vi "LeddarRead.vi"(9 "Frame Index":u32, 10 "Connection Mode":enum32{"INIT_FILE", "INIT_LIVE"}(radio), 11 "DeviceControl":refnum<k24>) -> (1 "New Status":bool, 2 "Detections Array":refnum<k24>[](array[refnum]), 3 "DeviceControl Out":refnum<k24>)   [LabVIEW 2012]
uses:
  C:/Program Files/LeddarTech/xtec/LeddarNET2.dll
  Globals.vi
panel:
  out "Timer value":dbl
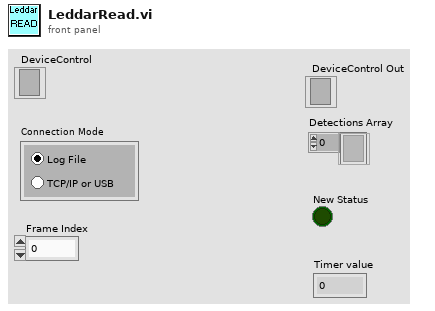
[diagram p1: front panel]
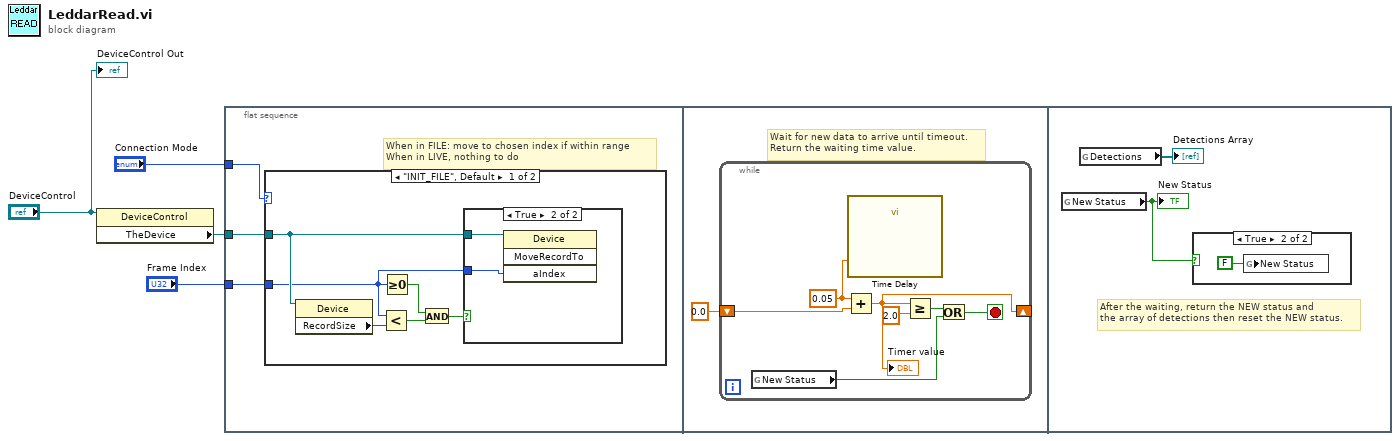
[diagram p0: block diagram]
diagram:
  n1 = property class="DeviceControl"(reference="DeviceControl") -> ("TheDevice"=w2:refnum<k24>)  [unwired: 1 in, 2 out]
  n2 = flat-sequence {
    tunnel: "Connection Mode" -> [w7]
    tunnel: w2 -> [w6]
    tunnel: "Frame Index" -> [w5]
    frame #0 {
      # "When in FILE: move to chosen index if within range\nWhen in LIVE, nothing to do"
      n3 = case shown="\"INIT_FILE\", Default" w7 {
        tunnel: w6 -> [w10 _]
        tunnel: w5 -> [w9 _]
        frame "INIT_FILE", Default {
          n4 = property class="Device"(reference=w10) -> ("RecordSize"=w8:u32)  [unwired: 1 in, 2 out]
          n5 = Less?(x=w9, y=w8) -> (x < y?=w13:bool)
          n6 = Greater Or Equal To 0?(x=w9) -> (x >= 0?=w12:bool)
          n7 = And(x=w12, y=w13) -> (x .and. y?=w11:bool)
          n8 = case shown="True" w11 {
            tunnel: w10 -> [_ w15]
            tunnel: w9 -> [_ w14]
            frame False {
            }
            frame True {
              n9 = invoke class="Device" method="MoveRecordTo"(reference=w15, "aIndex"=w14) -> ()  [unwired: 2 in, 4 out]
            }
          }
        }
        frame "INIT_LIVE" {
        }
      }
    }
    frame #1 {
      # "Wait for new data to arrive until timeout.\nReturn the waiting time value."
      n10 = while {
        shift-right: [w17] -> _
        shift-left: 0.0 ("y") -> [w21]
        stop <- w18 stop-if-true
        w20 = 0.05 ("Delay Time (s)")
        n11 = global read "Globals.vi" "New Status"() -> (w23:bool)
        n12 = Add(x=w20, y=w21) -> (x+y=w17:dbl)
        "Timer value" <- w17
        n13 = call "Time Delay"("Delay Time (s)"=w20) -> ()  [unwired: 10 in, 1 out]
        n14 = Greater Or Equal?(x=w17, y=2.0) -> (x >= y?=w19:bool)
        n15 = Or(x=w19, y=w23) -> (x .or. y?=w18:bool)
      }
    }
    frame #2 {
      # "After the waiting, return the NEW status and\nthe array of detections then reset the NEW status."
      n16 = global read "Globals.vi" "New Status"() -> (w24:bool)
      "New Status" <- w24
      n17 = global read "Globals.vi" "Detections"() -> (→"Detections Array":refnum<k24>[])
      n18 = case shown="True" w24 {
        frame False {
        }
        frame True {
          n19 = global write "Globals.vi" "New Status"(FALSE) -> ()
        }
      }
    }
  }
  "DeviceControl Out" <- "DeviceControl"
